vi "SLAM_Dispenser.vi"() -> ()   [LabVIEW 2012]
uses:
  <vilib>/DAQmx/read.llb/DAQmx Read.vi
  <vilib>/DAQmx/read.llb/DAQmx Read (Digital 1D Bool NChan 1Samp 1Line).vi
  <vilib>/DAQmx/write.llb/DAQmx Write.vi
  <vilib>/DAQmx/write.llb/DAQmx Write (Digital 1D Bool NChan 1Samp 1Line).vi
  <vilib>/DAQmx/configure/task.llb/DAQmx Clear Task.vi
  <vilib>/DAQmx/create/task.llb/DAQmx Create Task.vi
  <vilib>/DAQmx/configure/task.llb/DAQmx Start Task.vi
  <vilib>/DAQmx/create/channels.llb/DAQmx Create Virtual Channel.vi
  <vilib>/DAQmx/create/channels.llb/DAQmx Create Channel (DO-Digital Output).vi
  <vilib>/DAQmx/miscellaneous.llb/DAQmx Fill In Error Info.vi
  <vilib>/DAQmx/create/channels.llb/DAQmx Create Channel (DI-Digital Input).vi
panel:
  in  "Enable [B]":bool
  in  "Enable [A]":bool
  in  "Start Dispense Manual [B]":bool
  out "Test Display B":string="Mode: OFF  (Press Start to Begin)\r\r\r    "
  in  "Start Dispense Manual [A]":bool
  out "B Digital Output":bool[](array[boolean])
  out "Test Display A":string="Mode: OFF  (Press Start to Begin)\r\r\r    "
  out "A Digital Outputs":bool[](array[boolean])
  in  "ECOLAB Button":bool
  in  "Tab Control":enum32{"SYSTEM CONFIG", "CONFIG A", "CONFIG B"}(tab)
  in  "daq wait [ms]":u32
  in  "9485 Manual Control":bool[](array[boolean])=[FALSE, FALSE, FALSE, FALSE, FALSE, FALSE, FALSE, FALSE]
  in  "ON PULSE [s]":dbl=0.5
  in  "OFF PULSE [s]":dbl=0.5
  in  "Test Folder":path=path "C:/Users/ottinbr/Desktop"
  out "Test A Error":errorcluster
  out "Test B Error":errorcluster
  out "9481 0 Error":errorcluster
  out "DAQ Digital Loop":i32=12359
  out "MAIN Loop A":i32=12319
  out "MAIN Loop B":i32=12294
  out "9472 Error":errorcluster
  in  "9472 Name":tag="9472"
  in  "9472 Manual Control":bool[](array[boolean])=[FALSE, FALSE, FALSE, FALSE, FALSE, FALSE, FALSE, FALSE]
  in  "9411 Name":tag="9411"
  out "9411 Error":errorcluster={"status"=TRUE, "code"=-201003, "source"="DAQmx Create Channel (DI-Digital Input).vi:5<append>\n<B>Device Specified: </B>9411\n\n<B>Task Name: </B>9411"}
  in  "b wait [ms]":u32
  in  "a wait [ms]":u32
  out "Digital Inputs":bool[](array[boolean])
  out "9485":bool[](array[boolean])
  in  "9481 Name [0]":tag="9481"
  in  "9481 Name [1]":tag="9481"
  out "9481 1 Error":errorcluster
  in  "Test Cluster A":T1={"Load Test"=1, "New Test Name"="", "Test Description"="Default Dispense", "Step Select"=0, "Save Test"=FALSE, "Erase Test"=FALSE, "Max Steps"=7, "Loop Limit"=5, "Continue at Loop Limit?"=FALSE, "Step N"=2, "Test Array (Standard)"=[{"Step Number"=0, "Step Description"="Initialize", "Step Time Target"=0.5, "Step Time Unit"=0, "Step End Action"=0}, {"Step Number"=1, "Step Description"="H2O ON", "Step Time Target"=1.0, "Step Time Unit"=0, "Step End Action"=0}, {"Step Number"=2, "Step Description"="H2O OFF, Soap ON", "Step Time Target"=4.0, "Step Time Unit"=0, "Step End Action"=0}, {"Step Number"=3, "Step Description"="Scrub Delay Time", "Step Time Target"=4.0, "Step Time Unit"=0, "Step End Action"=0}, {"Step Number"=4, "Step Description"="Rinse Time", "Step Time Target"=20.0, "Step Time Unit"=0, "Step End Action"=0}, {"Step Number"=5, "Step Description"="Signal Complete", "Step Time Target"=1.5, "Step Time Unit"=0, "Step End Action"=0}, {"Step Number"=6, "Step Description"="Dispense Done", "Step Time Target"=0.5, "Step Time Unit"=0, "Step End Action"=65535}], "Test Array (Custom)"=[{"Digital Outputs"=[FALSE, FALSE, FALSE, FALSE, FALSE, FALSE, FALSE, FALSE]}, {"Digital Outputs"=[TRUE, TRUE, FALSE, FALSE, FALSE, FALSE, FALSE, FALSE]}, {"Digital Outputs"=[FALSE, TRUE, TRUE, FALSE, FALSE, FALSE, FALSE, FALSE]}, {"Digital Outputs"=[FALSE, FALSE, FALSE, TRUE, FALSE, FALSE, FALSE, FALSE]}, {"Digital Outputs"=[TRUE, FALSE, FALSE, FALSE, TRUE, TRUE, FALSE, FALSE]}, {"Digital Outputs"=[FALSE, FALSE, FALSE, FALSE, FALSE, FALSE, TRUE, FALSE]}, {"Digital Outputs"=[FALSE, FALSE, FALSE, FALSE, FALSE, FALSE, FALSE, FALSE]}]} {"Test Array (Standard)"."Step End Action" items=["Go to Next Step", "Loop to Step 0", "Loop to Step N", "Stop Test Mode", "Stop Program"]; "Test Array (Standard)"."Step Time Unit" items=["sec", "min", "hr"]; "Test Array (Standard)"."Step Time Target" min=0.001 format="%#.3f"; "Test Array (Standard)"."Step Number" min=0 step=1; "Load Test" items=["default", "Dispense_Default"]; "Step Select" step=1}
  out "A Digital Output Display":bool[](array[boolean])
  out "B Digital Output Display":bool[](array[boolean])
  in  "Test Cluster B":T1={"Load Test"=1, "New Test Name"="", "Test Description"="Default Dispense", "Step Select"=0, "Save Test"=FALSE, "Erase Test"=FALSE, "Max Steps"=7, "Loop Limit"=5, "Continue at Loop Limit?"=FALSE, "Step N"=2, "Test Array (Standard)"=[{"Step Number"=0, "Step Description"="Initialize", "Step Time Target"=0.5, "Step Time Unit"=0, "Step End Action"=0}, {"Step Number"=1, "Step Description"="H2O ON", "Step Time Target"=1.0, "Step Time Unit"=0, "Step End Action"=0}, {"Step Number"=2, "Step Description"="H2O OFF, Soap ON", "Step Time Target"=4.0, "Step Time Unit"=0, "Step End Action"=0}, {"Step Number"=3, "Step Description"="Scrub Delay Time", "Step Time Target"=4.0, "Step Time Unit"=0, "Step End Action"=0}, {"Step Number"=4, "Step Description"="Rinse Time", "Step Time Target"=20.0, "Step Time Unit"=0, "Step End Action"=0}, {"Step Number"=5, "Step Description"="Signal Complete", "Step Time Target"=1.5, "Step Time Unit"=0, "Step End Action"=0}, {"Step Number"=6, "Step Description"="Dispense Done", "Step Time Target"=0.5, "Step Time Unit"=0, "Step End Action"=65535}], "Test Array (Custom)"=[{"Digital Outputs"=[FALSE, FALSE, FALSE, FALSE, FALSE, FALSE, FALSE, FALSE]}, {"Digital Outputs"=[TRUE, TRUE, FALSE, FALSE, FALSE, FALSE, FALSE, FALSE]}, {"Digital Outputs"=[FALSE, TRUE, TRUE, FALSE, FALSE, FALSE, FALSE, FALSE]}, {"Digital Outputs"=[FALSE, FALSE, FALSE, TRUE, FALSE, FALSE, FALSE, FALSE]}, {"Digital Outputs"=[TRUE, FALSE, FALSE, FALSE, TRUE, TRUE, FALSE, FALSE]}, {"Digital Outputs"=[FALSE, FALSE, FALSE, FALSE, FALSE, FALSE, TRUE, FALSE]}, {"Digital Outputs"=[FALSE, FALSE, FALSE, FALSE, FALSE, FALSE, FALSE, FALSE]}]} {"Test Array (Standard)"."Step End Action" items=["Go to Next Step", "Loop to Step 0", "Loop to Step N", "Stop Test Mode", "Stop Program"]; "Test Array (Standard)"."Step Time Unit" items=["sec", "min", "hr"]; "Test Array (Standard)"."Step Time Target" min=0.001 format="%#.3f"; "Test Array (Standard)"."Step Number" min=0 step=1; "Load Test" items=["default", "Dispense_Default"]; "Step Select" step=1}
  in  "Stop Program":bool=TRUE
  # "ENABLE DISP"
  # "MANUAL START"
  # "Created by Blake Otting\nSystems Engineering Lab\n2-13-2013"
  # "Project SLAM:  Dispenser Test"
  # "H20 GRN [A]"
  # "H20 VLV [A]"
  # "Scrub GRN [A]"
  # "SOAP [A]"
  # "Rinse GRN [A]"
  # "VLV STATE [A]"
  # "RED [A]"
  # "H20 VLV [B]"
  # "SOAP [B]"
  # "H20 GRN [B]"
  # "VLV STATE [B]"
  # "Scrub GRN [B]"
  # "EXTRA [A]"
  # "Rinse GRN [B]"
  # "RED [B]"
  # "EXTRA [B]"
  # "Extra"
  # "Red LED's"
  # "Rinse Green LED"
  # "+1 on Hand Remove"
  # "Scrub Green LED"
  # "Soap Control"
  # "Water Green LED"
  # "H2O Control"
  # "Scroll"
  # "Step"
  # "Description"
  # "Time Target"
  # "End Action"
  # "Total #\nof Steps"
  # "Extra"
  # "Red LED's"
  # "Rinse Green LED"
  # "+1 on Hand Remove"
  # "Scrub Green LED"
  # "Soap Control"
  # "Water Green LED"
  # "H2O Control"
  # "Scroll"
  # "Step"
  # "Description"
  # "Time Target"
  # "End Action"
  # "Total #\nof Steps"
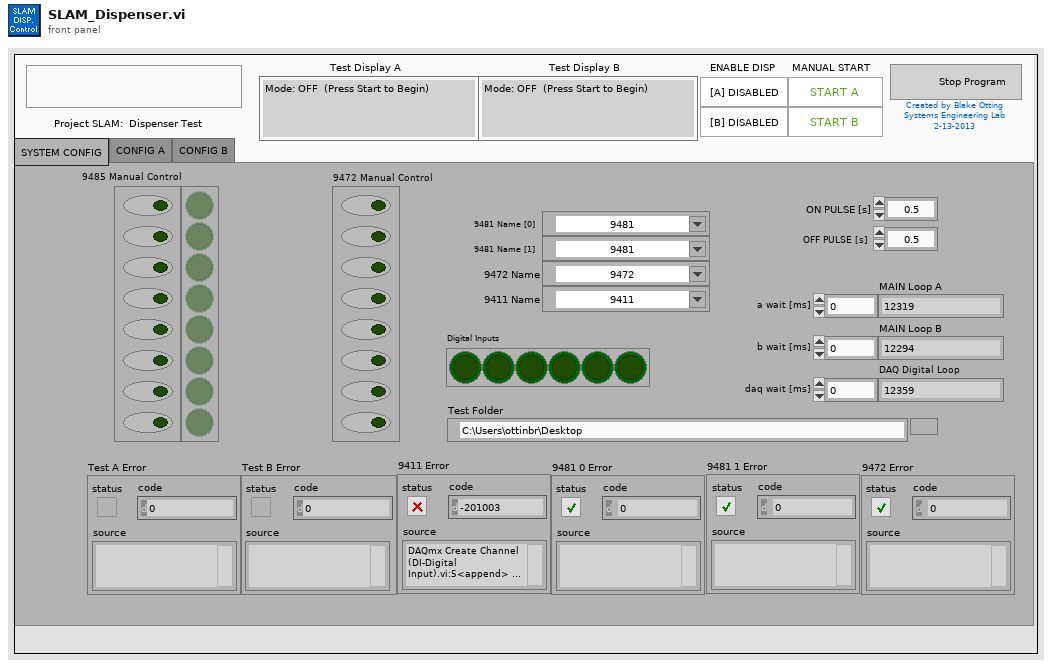
[diagram p1: front panel]
types:
  T1 = cluster{"Load Test":u16, "New Test Name":string, "Test Description":string, "Step Select":u16, "Save Test":bool, "Erase Test":bool, "Max Steps":u16, "Loop Limit":u16, "Continue at Loop Limit?":bool, "Step N":u16, "Test Array (Standard)":cluster{"Step Number":i32, "Step Description":string, "Step Time Target":dbl, "Step Time Unit":u16, "Step End Action":u16}[], "Test Array (Custom)":cluster{"Digital Outputs":bool[]}[]}
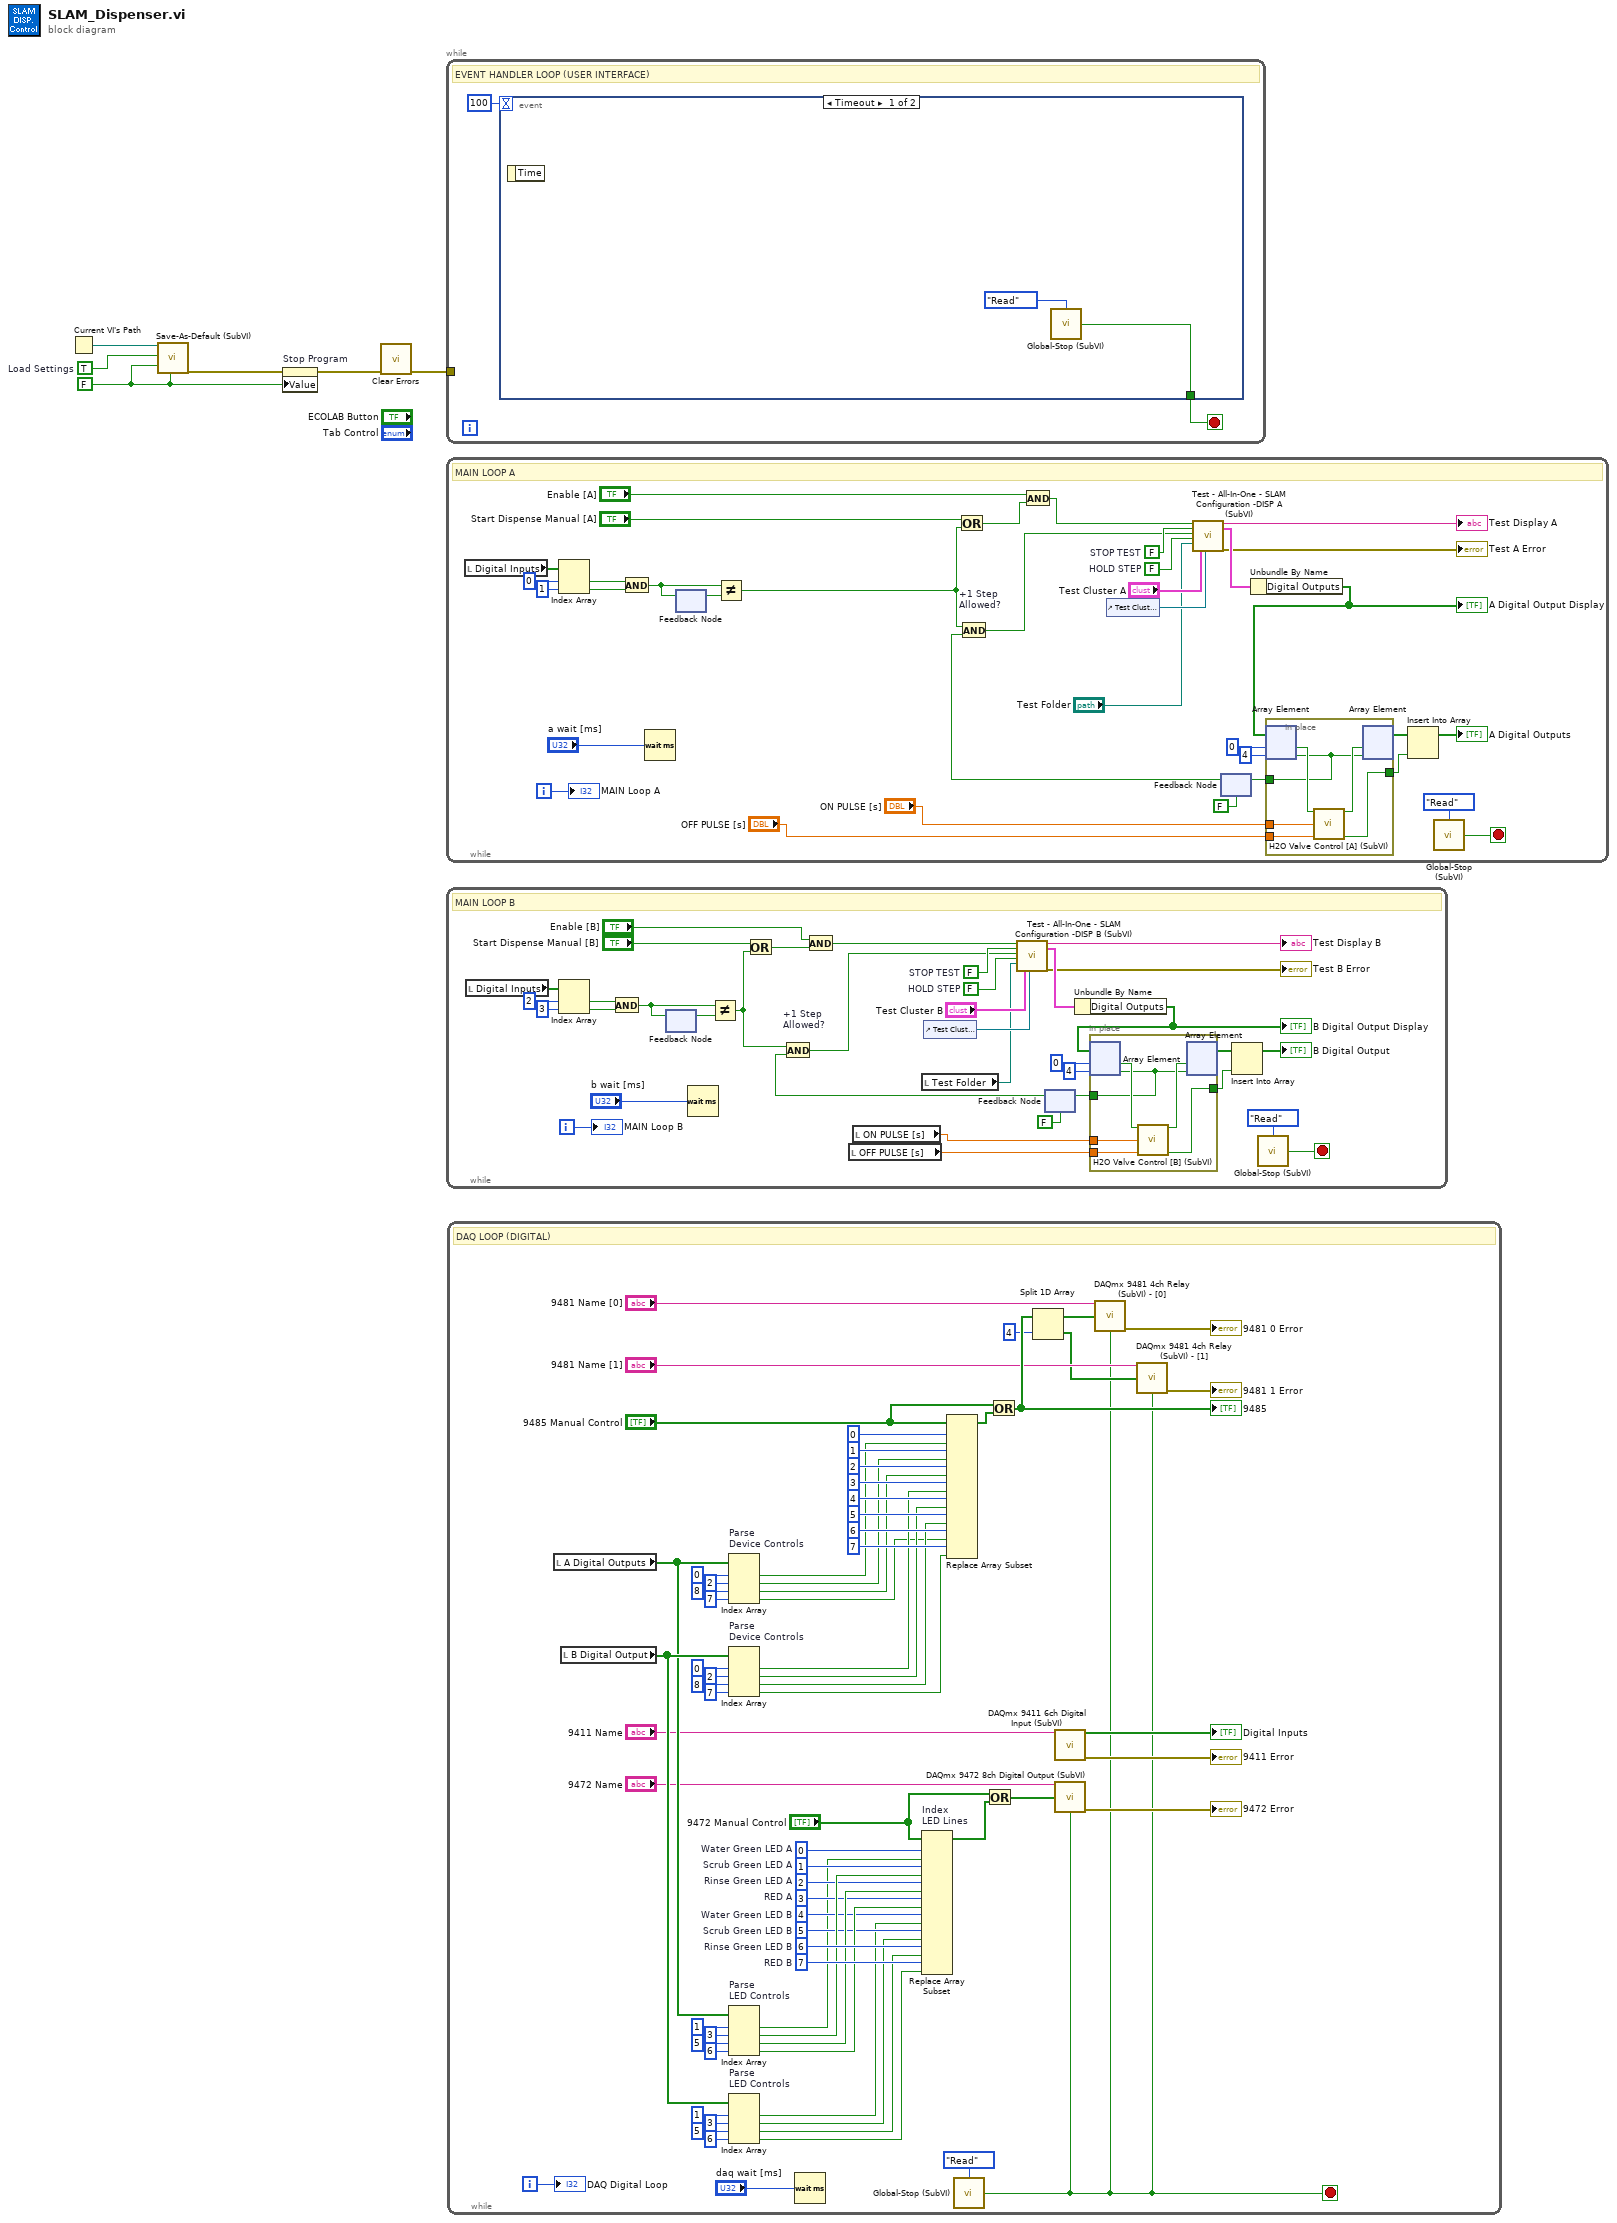
[diagram p0: block diagram]
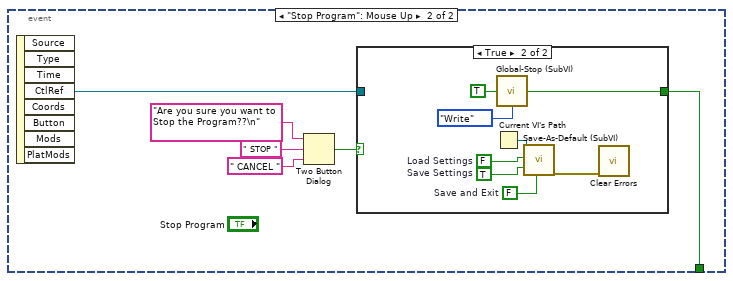
[diagram p2: hidden frame]
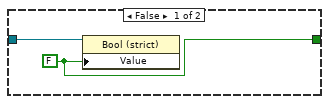
[diagram p3: hidden frame]
diagram:
  w3 = TRUE  # Load Settings
  w1 = FALSE
  n1 = Current VI's Path() -> (path=w4:path)
  n2 = call "Save-As-Default (SubVI).vi"("Current VI's Path"=w4, "Load Settings"=w3, "Save Settings"=w1, "Save and Exit"=w1) -> ("Save as Default Error"=w2:errorcluster)  [unwired: 15 in]
  n3 = property on="Stop Program" class="Bool (strict)"(error in=w2, "Value"=w1) -> (error out=w6:errorcluster)  [unwired: 1 in, 1 out]
  n4 = call <vilib>:"Clear Errors.vi"("error in (no error)"=w6) -> ("error out"=w5:errorcluster)  [unwired: 6 out]
  n5 = while {
    tunnel: w5 -> [_]
    stop <- w8 stop-if-true
    # "EVENT HANDLER LOOP (USER INTERFACE)"
    n6 = event shown="[0] Timeout" {
      selector: _ -> [_ _]
      dyn-events: _ -> [_ _]
      timeout: 100 -> [_ _]
      tunnel: [w9 w12] -> w8
      event Timeout {
        n7 = event-data() -> ()  [unwired: 2 out]
        n8 = call "Global-Stop (SubVI).vi"("Mode (Read)"=enum16{"Read", "Write"}."Read") -> ("OUT"=w9:bool)  [unwired: 3 in]
      }
      event "Stop Program": Mouse Up {
        n9 = event-data() -> ("CtlRef"=w11:refnum<vi>)  [unwired: 8 out]
        n10 = Two Button Dialog(message="Are you sure you want to Stop the Program??\n", 1:" CANCEL " ("F button name (\"Cancel\")"), 2:" STOP ") -> (T button?=w13:bool)
        n11 = case shown="True" w13 {
          tunnel: [w17 w24] -> w12
          tunnel: w11 -> [w18 _]
          frame False {
            w17 = FALSE ("Value")
            n12 = property class="Bool (strict)"(reference=w18, "Value"=w17) -> ()  [unwired: 1 in, 2 out]
          }
          frame True {
            w20 = FALSE  # Save and Exit
            w21 = TRUE  # Save Settings
            w22 = FALSE  # Load Settings
            n13 = Current VI's Path() -> (path=w23:path)
            n14 = call "Global-Stop (SubVI).vi"("Mode (Read)"=enum16{"Read", "Write"}."Write", "IN"=TRUE) -> ("OUT"=w24:bool)  [unwired: 2 in]
            n15 = call "Save-As-Default (SubVI).vi"("Current VI's Path"=w23, "Load Settings"=w22, "Save Settings"=w21, "Save and Exit"=w20) -> ("Save as Default Error"=w19:errorcluster)  [unwired: 15 in]
            n16 = call <vilib>:"Clear Errors.vi"("error in (no error)"=w19) -> ()  [unwired: 7 out]
          }
        }
      }
    }
  }
  n17 = while {
    i -> [w60]
    stop <- w61 stop-if-true
    w51 = FALSE  # STOP TEST
    w43 = FALSE  # HOLD STEP
    # "MAIN LOOP A"
    n18 = local read "Digital Inputs"() -> (w39:bool[])
    n19 = Index Array(array=w39, index #1=0, index #2=1) -> (element #1=w36:bool, element #2=w35:bool)
    n20 = And(x=w36, y=w35) -> (x .and. y?=w37:bool)
    n21 = Wait (ms)(milliseconds to wait="a wait [ms]") -> ()  [unwired: 1 out]
    n22 = feedback #1() -> (w38:bool)  [unwired: 1 in]
    n23 = feedback-in #1(w37) -> ()
    n24 = Not Equal?(x=w37, y=w38) -> (x != y?=w33:bool)
    n25 = Or(x="Start Dispense Manual [A]", y=w33) -> (x .or. y?=w32:bool)
    n26 = And(x="Enable [A]", y=w32) -> (x .and. y?=w30:bool)
    n27 = control-ref of="Test Cluster A"() -> (w58:refnum<vi>)
    n28 = feedback #2(FALSE) -> (w47:bool)
    n29 = And "+1 Step\nAllowed?"(x=w33, y=w47) -> (x .and. y?=w44:bool)
    n30 = call "Test - All-In-One - SLAM Configuration -DISP A (SubVI).vi"("START TEST"=w30, "STOP TEST"=w51, "NEXT STEP"=w44, "HOLD STEP"=w43, "Test Folder"="Test Folder", "SLAM Test Cluster"="Test Cluster A", "SLAM Test Cluster Ref"=w58) -> ("Test Display"=→"Test Display A":string, "Test Output"=w57:cluster{"Digital Outputs":bool[]}, "Error Output"=→"Test A Error":errorcluster)  [unwired: 5 in, 5 out]
    n31 = Unbundle By Name(w57) -> ("Digital Outputs"=w49:bool[])
    "A Digital Output Display" <- w49
    n32 = in-place {
      in-place-border: [w66] -> w54
      in-place-border: "ON PULSE [s]" -> [w65]
      in-place-border: "OFF PULSE [s]" -> [w64]
      in-place-border: [w63] -> w46
      n33 = in-place-array #3(w49, 0, 4) -> (w68:bool, w63:bool)
      n34 = call "H2O Valve Control [A] (SubVI).vi"("Water Valve Command"=w68, "ON PULSE"=w65, "OFF PULSE"=w64) -> ("H2O Valve Signal"=w67:bool, "H2O Valve Reverse"=w66:bool)  [unwired: 10 in, 1 out]
      n35 = in-place-array #3(w67, w63) -> (w55:bool[])  [unwired: 2 out]
    }
    n36 = feedback-in #2(w46) -> ()
    n37 = Insert Into Array(array=w55, new element=w54) -> (→"A Digital Outputs":bool[])  [unwired: 1 in]
    n38 = call "Global-Stop (SubVI).vi"("Mode (Read)"=enum16{"Read", "Write"}."Read") -> ("OUT"=w61:bool)  [unwired: 3 in]
    "MAIN Loop A" <- w60
  }
  n39 = while {
    i -> [w102]
    stop <- w103 stop-if-true
    w96 = FALSE  # STOP TEST
    w89 = FALSE  # HOLD STEP
    # "MAIN LOOP B"
    n40 = local read "Digital Inputs"() -> (w83:bool[])
    n41 = Index Array(array=w83, index #1=2, index #2=3) -> (element #1=w82:bool, element #2=w81:bool)
    n42 = And(x=w82, y=w81) -> (x .and. y?=w79:bool)
    n43 = feedback #4() -> (w80:bool)  [unwired: 1 in]
    n44 = feedback-in #4(w79) -> ()
    n45 = Wait (ms)(milliseconds to wait="b wait [ms]") -> ()  [unwired: 1 out]
    n46 = Not Equal?(x=w79, y=w80) -> (x != y?=w78:bool)
    n47 = Or(x="Start Dispense Manual [B]", y=w78) -> (x .or. y?=w73:bool)
    n48 = And(x="Enable [B]", y=w73) -> (x .and. y?=w72:bool)
    n49 = local read "OFF PULSE [s]"() -> (w69:dbl)
    n50 = local read "ON PULSE [s]"() -> (w70:dbl)
    n51 = local read "Test Folder"() -> (w71:path)
    n52 = control-ref of="Test Cluster B"() -> (w76:refnum<vi>)
    n53 = feedback #5(FALSE) -> (w93:bool)
    n54 = And "+1 Step\nAllowed?"(x=w78, y=w93) -> (x .and. y?=w90:bool)
    n55 = call "Test - All-In-One - SLAM Configuration -DISP B (SubVI).vi"("START TEST"=w72, "STOP TEST"=w96, "NEXT STEP"=w90, "HOLD STEP"=w89, "Test Folder"=w71, "SLAM Test Cluster"="Test Cluster B", "SLAM Test Cluster Ref"=w76) -> ("Test Display"=→"Test Display B":string, "Test Output"=w101:cluster{"Digital Outputs":bool[]}, "Error Output"=→"Test B Error":errorcluster)  [unwired: 5 in, 5 out]
    n56 = Unbundle By Name(w101) -> ("Digital Outputs"=w85:bool[])
    "B Digital Output Display" <- w85
    n57 = in-place {
      in-place-border: [w108] -> w98
      in-place-border: w70 -> [w107]
      in-place-border: w69 -> [w106]
      in-place-border: [w105] -> w92
      n58 = in-place-array #6(w85, 0, 4) -> (w110:bool, w105:bool)
      n59 = call "H2O Valve Control [B] (SubVI).vi"("Water Valve Command"=w110, "ON PULSE"=w107, "OFF PULSE"=w106) -> ("H2O Valve Signal"=w109:bool, "H2O Valve Reverse"=w108:bool)  [unwired: 10 in, 1 out]
      n60 = in-place-array #6(w109, w105) -> (w99:bool[])  [unwired: 2 out]
    }
    n61 = feedback-in #5(w92) -> ()
    n62 = Insert Into Array(array=w99, new element=w98) -> (→"B Digital Output":bool[])  [unwired: 1 in]
    n63 = call "Global-Stop (SubVI).vi"("Mode (Read)"=enum16{"Read", "Write"}."Read") -> ("OUT"=w103:bool)  [unwired: 3 in]
    "MAIN Loop B" <- w102
  }
  n64 = while {
    i -> [w173]
    stop <- w111 stop-if-true
    w171 = 7  # RED B
    w170 = 6  # Rinse Green LED B
    w166 = 5  # Scrub Green LED B
    w165 = 4  # Water Green LED B
    w164 = 3  # RED A
    w163 = 2  # Rinse Green LED A
    w162 = 1  # Scrub Green LED A
    w161 = 0  # Water Green LED A
    # "DAQ LOOP (DIGITAL)"
    n65 = local read "A Digital Outputs"() -> (w144:bool[])
    n66 = local read "B Digital Output"() -> (w156:bool[])
    n67 = Index Array "Parse\nDevice Controls"(array=w144, index #1=0, index #2=2, index #3=8, index #4=7) -> (element #1=w127:bool, element #2=w147:bool, element #3=w148:bool, element #4=w120:bool)
    n68 = Index Array "Parse\nDevice Controls"(array=w156, index #1=0, index #2=2, index #3=8, index #4=7) -> (element #1=w157:bool, element #2=w158:bool, element #3=w159:bool, element #4=w121:bool)
    n69 = Index Array "Parse\nLED Controls"(array=w144, index #1=1, index #2=3, index #3=5, index #4=6) -> (element #1=w160:bool, element #2=w169:bool, element #3=w168:bool, element #4=w167:bool)
    n70 = Index Array "Parse\nLED Controls"(array=w156, index #1=1, index #2=3, index #3=5, index #4=6) -> (element #1=w136:bool, element #2=w135:bool, element #3=w134:bool, element #4=w133:bool)
    n71 = Wait (ms)(milliseconds to wait="daq wait [ms]") -> ()  [unwired: 1 out]
    n72 = Replace Array Subset "Index\nLED Lines"(array="9472 Manual Control", new element #1=w160, index #1=w161, new element #2=w169, index #2=w162, new element #3=w168, index #3=w163, new element #4=w167, index #4=w164, new element #5=w136, index #5=w165, new element #6=w135, index #6=w166, new element #7=w134, index #7=w170, new element #8=w133, index #8=w171) -> (w129:bool[])
    n73 = Replace Array Subset(array="9485 Manual Control", new element #1=w127, index #1=0, new element #2=w147, index #2=1, new element #3=w148, index #3=2, new element #4=w157, index #4=3, new element #5=w158, index #5=4, new element #6=w159, index #6=5, new element #7=w120, index #7=6, new element #8=w121, index #8=7) -> (w146:bool[])
    n74 = call "Global-Stop (SubVI).vi"("Mode (Read)"=enum16{"Read", "Write"}."Read") -> ("OUT"=w111:bool)  [unwired: 3 in]
    n75 = Or(x="9472 Manual Control", y=w129) -> (x .or. y?=w128:bool[])
    n76 = Or(x="9485 Manual Control", y=w146) -> (x .or. y?=w119:bool[])
    "9485" <- w119
    n77 = Split 1D Array(array=w119, index=4) -> (first subarray=w116:bool[], second subarray=w113:bool[])
    n78 = call "DAQmx 9411 6ch Digital Input (SubVI).vi"("9411 Name"="9411 Name") -> ("Digital Inputs"=→"Digital Inputs":bool[], "9411 Error"=→"9411 Error":errorcluster)  [unwired: 13 in]
    n79 = call "DAQmx 9472 8ch Digital Output (SubVI).vi"("9472 Name"="9472 Name", "Output Control"=w128, "Stop Program"=w111) -> ("9472 Error"=→"9472 Error":errorcluster)  [unwired: 12 in]
    n80 = call "DAQmx 9481 4ch Relay (SubVI) - [0].vi"("9481 Name"="9481 Name [0]", "Relay Control"=w116, "Stop Program"=w111) -> ("9481 Error"=→"9481 0 Error":errorcluster)  [unwired: 12 in]
    n81 = call "DAQmx 9481 4ch Relay (SubVI) - [1].vi"("9481 Name"="9481 Name [1]", "Relay Control"=w113, "Stop Program"=w111) -> ("9481 Error"=→"9481 1 Error":errorcluster)  [unwired: 12 in]
    "DAQ Digital Loop" <- w173
  }
